vi "Valve Control VI.vi"(7 "Boolean":bool, 8 "error in (no error)":errorcluster, 9 "B Valves":string, 10 "A Valves":string, 11 "VISA Refnum in":refnum<visa-resource-name>) -> (0 "error out":errorcluster, 3 "VISA Resource Name Out":refnum<visa-resource-name>)   [LabVIEW 2020]
uses:
  <instrlib>/Agilent 34970/Agilent 34970.lvlib
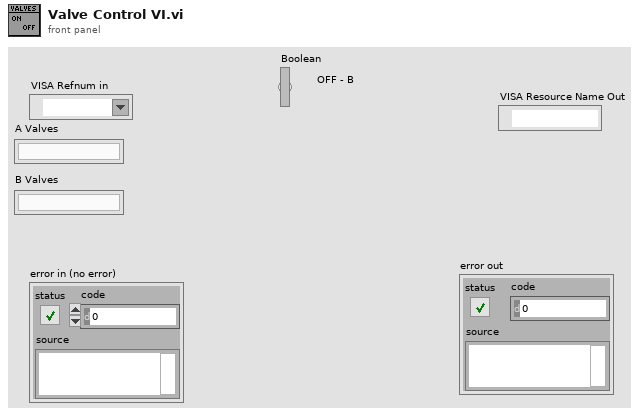
[diagram p1: front panel]
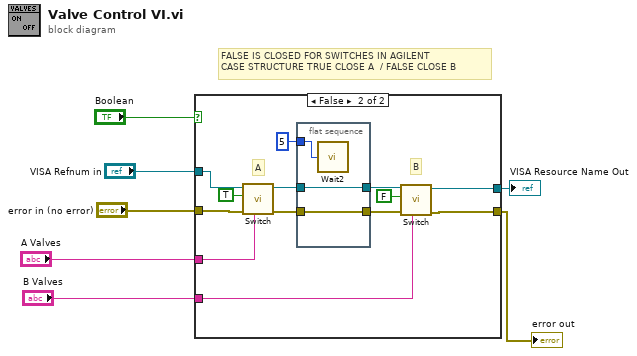
[diagram p0: block diagram]
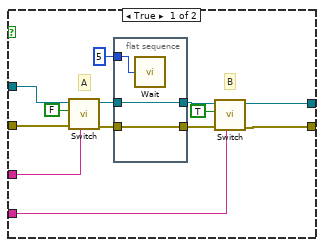
[diagram p2: hidden frame]
diagram:
  # "FALSE IS CLOSED FOR SWITCHES IN AGILENT\nCASE STRUCTURE TRUE CLOSE A  / FALSE CLOSE B"
  n1 = case shown="False" "Boolean" {
    tunnel: [w20 w36] -> w7
    tunnel: "error in (no error)" -> [w19 w35]
    tunnel: "VISA Refnum in" -> [w18 w34]
    tunnel: [w17 w33] -> w3
    tunnel: "A Valves" -> [w14 w30]
    tunnel: "B Valves" -> [w13 w29]
    frame True {
      # "B"
      # "A"
      n2 = call <instrlib>:"Switch.vi"("Channel List(empty)"=w14, "error in (no error)"=w19, "Open/Close (F:Close)"=FALSE, "VISA Resource Name"=w18) -> ("error out"=w10:errorcluster, "VISA Resource Name Out"=w12:refnum<visa-resource-name>)  [unwired: 5 in, 1 out]
      n3 = flat-sequence {
        tunnel: w12 -> [w23]
        tunnel: [w23] -> w11
        tunnel: [w22] -> w9
        tunnel: w10 -> [w22]
        tunnel: u32 5 ("Count(mSec)") -> [w21]
        frame #0 {
          n4 = call "Wait"("Count(mSec)"=w21) -> ()  [unwired: 1 out]
        }
      }
      n5 = call <instrlib>:"Switch.vi"("Channel List(empty)"=w13, "error in (no error)"=w9, "Open/Close (F:Close)"=TRUE, "VISA Resource Name"=w11) -> ("error out"=w20:errorcluster, "VISA Resource Name Out"=w17:refnum<visa-resource-name>)  [unwired: 5 in, 1 out]
    }
    frame False {
      # "B"
      # "A"
      n6 = call <instrlib>:"Switch.vi"("Channel List(empty)"=w30, "error in (no error)"=w35, "Open/Close (F:Close)"=TRUE, "VISA Resource Name"=w34) -> ("error out"=w26:errorcluster, "VISA Resource Name Out"=w27:refnum<visa-resource-name>)  [unwired: 5 in, 1 out]
      n7 = flat-sequence {
        tunnel: w27 -> [w39]
        tunnel: [w39] -> w24
        tunnel: [w38] -> w25
        tunnel: w26 -> [w38]
        tunnel: u32 5 ("Count(mSec)") -> [w37]
        frame #0 {
          n8 = call "Wait2"("Count(mSec)"=w37) -> ()  [unwired: 1 out]
        }
      }
      n9 = call <instrlib>:"Switch.vi"("Channel List(empty)"=w29, "error in (no error)"=w25, "Open/Close (F:Close)"=FALSE, "VISA Resource Name"=w24) -> ("error out"=w36:errorcluster, "VISA Resource Name Out"=w33:refnum<visa-resource-name>)  [unwired: 5 in, 1 out]
    }
  }
  "error out" <- w7
  "VISA Resource Name Out" <- w3
